vi "Wait on Delivery.vi"(8 "error in (no error)":errorcluster, 9 "Timeout (500)":u32=500, 10 "Delivery Notifier":refnum<notifier>, 11 "Sample Line in":refnum<class "Sample Line.lvclass">) -> (0 "error out":errorcluster, 3 "Sample Line out":refnum<class "Sample Line.lvclass">)   [LabVIEW 2015, in "cRIO-Carbondioxide.lvlib" / "CO2-Actor.lvlib" / "Sample Line.lvclass"]
uses:
  Sample Line.lvclass
  <vilib>/ActorFramework/Time-Delayed Send Message/Time-Delay Override Options.ctl
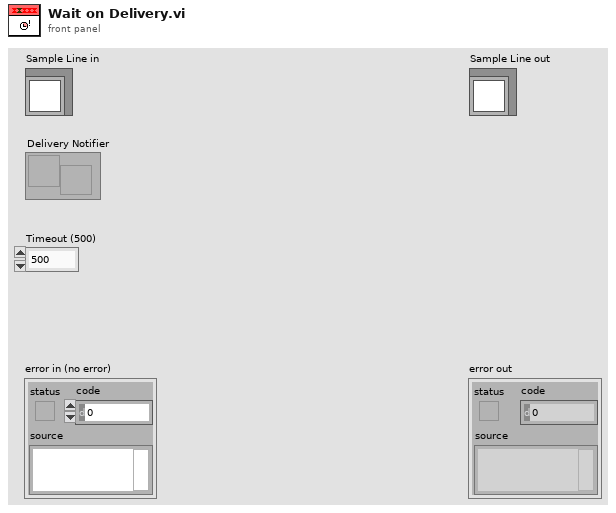
[diagram p1: front panel]
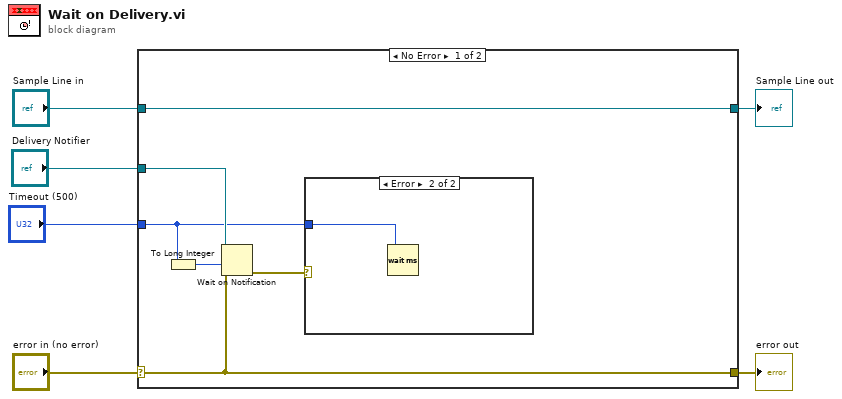
[diagram p0: block diagram]
diagram:
  n1 = case shown="No Error" "error in (no error)" {
    selector: "error in (no error)" -> [w10 w15]
    tunnel: [w10 w15] -> w5
    tunnel: [w12 w14] -> w3
    tunnel: "Sample Line in" -> [w12 w14]
    tunnel: "Timeout (500)" -> [w7 _]
    tunnel: "Delivery Notifier" -> [w11 _]
    frame No Error {
      n2 = To Long Integer(number=w7) -> (32bit integer=w9:i32)
      n3 = Wait on Notification(notifier=w11, timeout in ms (-1)=w9, error in (no error)=w10) -> (error out=w8:errorcluster)  [unwired: 1 in, 3 out]
      n4 = case shown="Error" w8 {
        tunnel: w7 -> [_ w13]
        frame No Error {
        }
        frame Error {
          n5 = Wait (ms)(milliseconds to wait=w13) -> ()  [unwired: 1 out]
        }
      }
    }
    frame Error {
    }
  }
  "error out" <- w5
  "Sample Line out" <- w3
